vi "STRINGhorafechA(SubVI).vi"() -> (0 "STRINGhora_fecha":string)   [LabVIEW 2015]
panel:
  out "date/time string":string
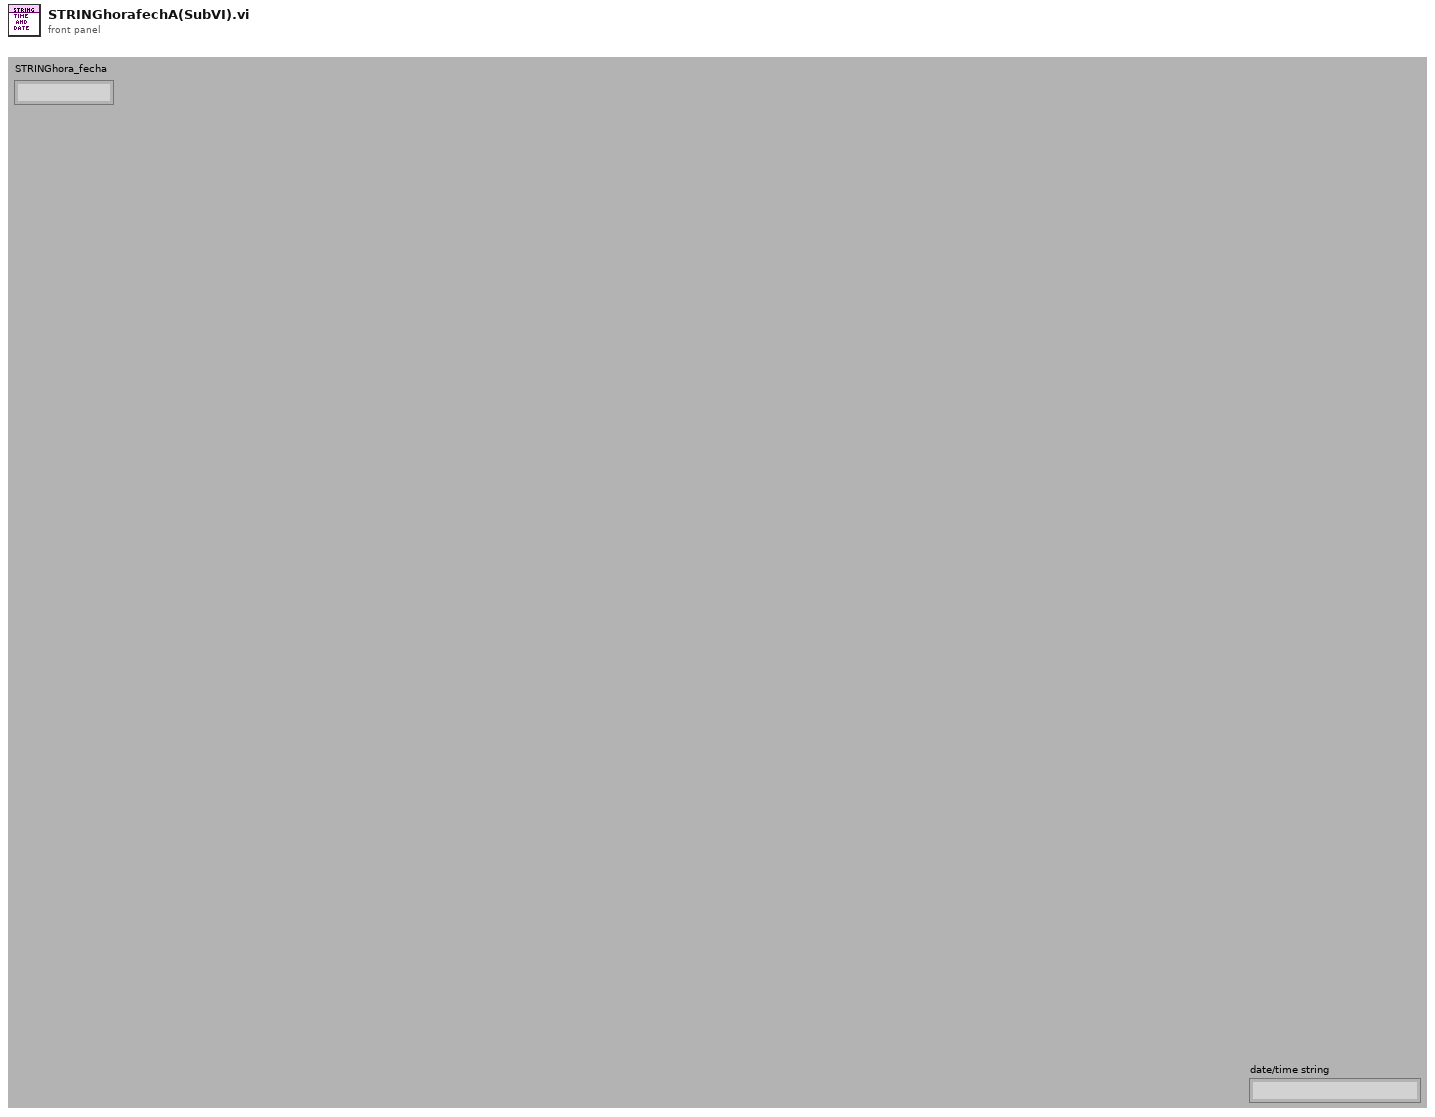
[diagram p1: front panel]
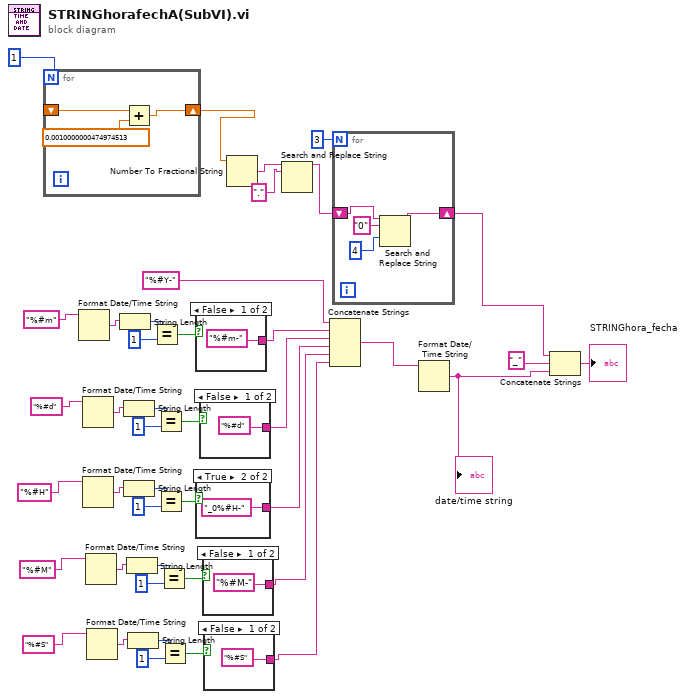
[diagram p0: block diagram]
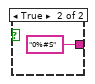
[diagram p2: hidden frame]
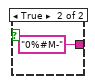
[diagram p3: hidden frame]
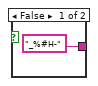
[diagram p4: hidden frame]
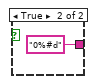
[diagram p5: hidden frame]
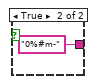
[diagram p6: hidden frame]
diagram:
  n1 = for {
    N: 1 -> [_]
    shift-right: [w45] -> w37
    shift-left: _ -> [w43]
    n2 = Add(x=w43, y=sgl 0.001) -> (x+y=w45:sgl)
  }
  n3 = Format Date/Time String(time format string (%c)="%#m") -> (date/time string=w24:string)  [unwired: 2 in]
  n4 = Format Date/Time String(time format string (%c)="%#d") -> (date/time string=w29:string)  [unwired: 2 in]
  n5 = Format Date/Time String(time format string (%c)="%#H") -> (date/time string=w17:string)  [unwired: 2 in]
  n6 = Format Date/Time String(time format string (%c)="%#M") -> (date/time string=w12:string)  [unwired: 2 in]
  n7 = Format Date/Time String(time format string (%c)="%#S") -> (date/time string=w7:string)  [unwired: 2 in]
  n8 = String Length(string=w24) -> (length=w25:i32)
  n9 = String Length(string=w29) -> (length=w30:i32)
  n10 = String Length(string=w17) -> (length=w18:i32)
  n11 = String Length(string=w12) -> (length=w13:i32)
  n12 = String Length(string=w7) -> (length=w8:i32)
  n13 = Equal?(x=w25, y=1) -> (x = y?=w27:bool)
  n14 = Equal?(x=w30, y=1) -> (x = y?=w32:bool)
  n15 = Equal?(x=w18, y=1) -> (x = y?=w20:bool)
  n16 = Equal?(x=w13, y=1) -> (x = y?=w15:bool)
  n17 = Equal?(x=w8, y=1) -> (x = y?=w10:bool)
  n18 = case shown="False" w27 {
    tunnel: ["%#m-" ("time format string (%c)") "0%#m-" ("time format string (%c)")] -> w34
    frame False {
    }
    frame True {
    }
  }
  n19 = case shown="True" w20 {
    tunnel: ["_%#H-" ("time format string (%c)") "_0%#H-" ("time format string (%c)")] -> w5
    frame False {
    }
    frame True {
    }
  }
  n20 = case shown="False" w32 {
    tunnel: ["%#d" ("time format string (%c)") "0%#d" ("time format string (%c)")] -> w35
    frame False {
    }
    frame True {
    }
  }
  n21 = case shown="False" w15 {
    tunnel: ["%#M-" ("time format string (%c)") "0%#M-" ("time format string (%c)")] -> w4
    frame False {
    }
    frame True {
    }
  }
  n22 = case shown="False" w10 {
    tunnel: ["%#S" ("time format string (%c)") "0%#S" ("time format string (%c)")] -> w3
    frame False {
    }
    frame True {
    }
  }
  n23 = Number To Fractional String(number=w37) -> (F-format string=w41:string)  [unwired: 3 out]
  n24 = Search and Replace String(input string=w41, search string="." ("replace string (\"\")")) -> (result string=w39:string)  [unwired: 1 in, 8 out]
  n25 = Concatenate Strings("%#Y-" ("time format string (%c)"), w34, w35, w5, w4, w3) -> (w36:string)
  n26 = for {
    N: 3 -> [_]
    shift-right: [w58] -> w2
    shift-left: w39 -> [w56]
    n27 = Search and Replace String(input string=w56, search string="0", offset=4 ("offset (0)")) -> (result string=w58:string)  [unwired: 1 in, 7 out]
  }
  n28 = Format Date/Time String(time format string (%c)=w36) -> (date/time string=w21:string)  [unwired: 2 in]
  "date/time string" <- w21
  n29 = Concatenate Strings(w2, "_" ("replace string (\"\")"), w21) -> (→"STRINGhora_fecha":string)
